vi "Activate ECL Guest Internet (SubVI).vi"(0 "Status String Ref":refnum<vi>, 7 "Activate":bool, 11 "Error IN":errorcluster, 14 "Ok to Click?":bool) -> (15 "Error OUT":errorcluster)   [LabVIEW 2012]
panel:
  in  "Web Browser":refnum<k7>(container)
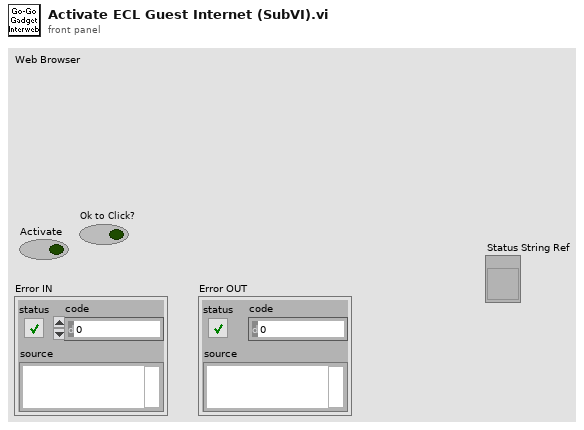
[diagram p1: front panel]
types:
  T1 = enum16{"Initialize", "Wait for Authorize Page", "Click Authorize", "Idle", "Exit"}
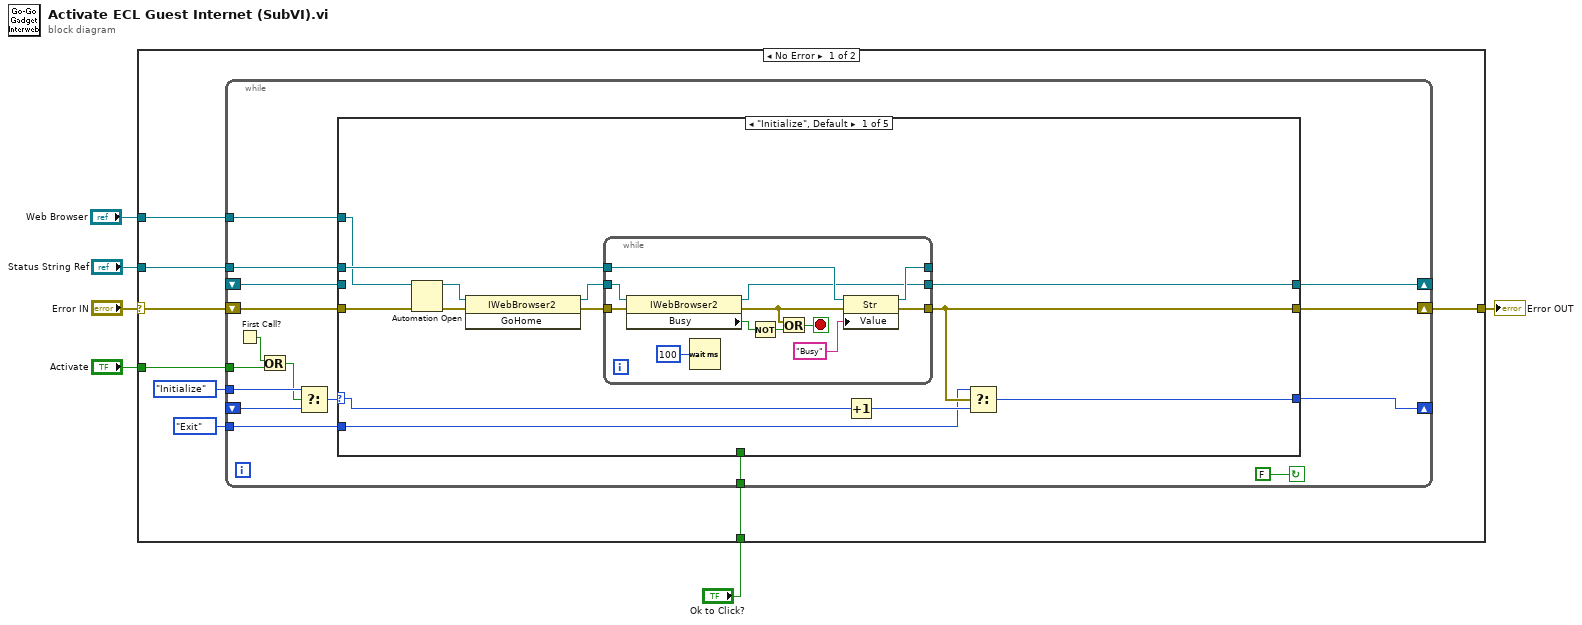
[diagram p0: block diagram]
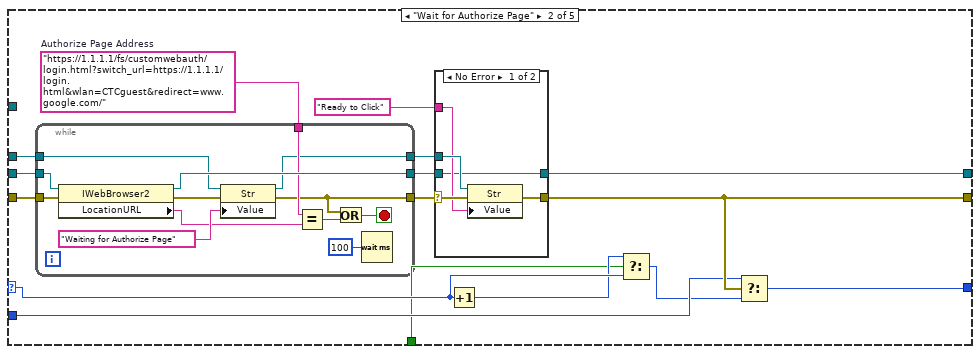
[diagram p2: hidden frame]
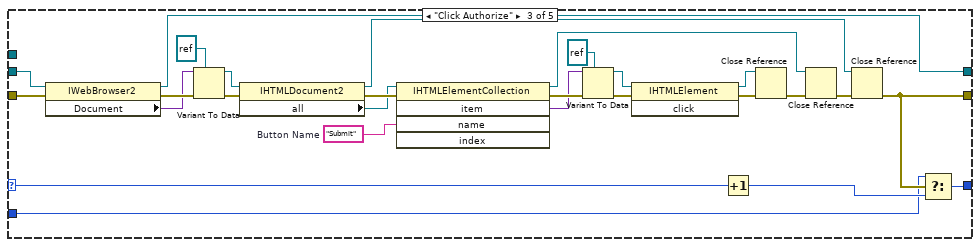
[diagram p4: hidden frame]
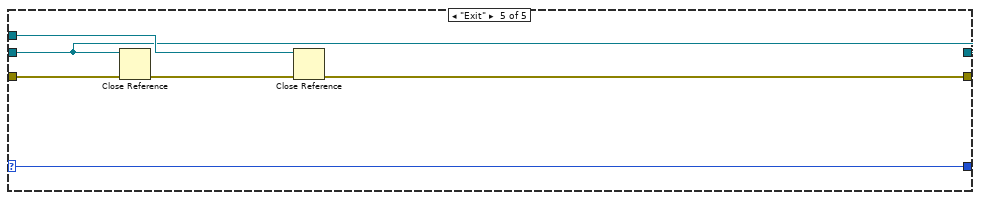
[diagram p6: hidden frame]
diagram:
  n1 = case shown="No Error" "Error IN" {
    selector: "Error IN" -> [w9 w128]
    tunnel: "Status String Ref" -> [w14 _]
    tunnel: "Activate" -> [w11 _]
    tunnel: [w10 w128] -> w4
    tunnel: "Web Browser" -> [w8 _]
    tunnel: "Ok to Click?" -> [w7 _]
    frame No Error {
      n2 = while {
        shift-right: [w29] -> _
        shift-left: _ -> [w28]
        shift-right: [w25] -> w10
        shift-left: w9 -> [w27]
        tunnel: w14 -> [w26]
        shift-right: [w21] -> _
        shift-left: _ -> [w23]
        tunnel: T1."Initialize" ("State") -> [w24]
        tunnel: T1."Exit" ("State") -> [w20]
        tunnel: w11 -> [w19]
        tunnel: w8 -> [w16]
        tunnel: w7 -> [w15]
        stop <- FALSE continue-if-true
        n3 = First Call?() -> (First Call?: T/F=w18:bool)
        n4 = Or(x=w18, y=w19) -> (x .or. y?=w17:bool)
        n5 = Select(t=w24, s=w17, f=w23) -> (s? t:f=w22:T1)
        n6 = case shown="\"Initialize\", Default" w22 {
          selector: w22 -> [w35 w59 w115 w121 w123]
          tunnel: [w37 w63 w116 w119 w122] -> w29
          tunnel: w28 -> [_ w70 w117 w119 w122]
          tunnel: w27 -> [w38 w71 w118 w120 w127]
          tunnel: w26 -> [w41 w69 _ _ w126]
          tunnel: [w36 w62 w113 w120 w124] -> w25
          tunnel: [w33 w60 w114 w121 w123] -> w21
          tunnel: w20 -> [w32 w61 w92 _ _]
          tunnel: w16 -> [w31 _ _ _ _]
          tunnel: w15 -> [_ w56 _ _ _]
          frame "Initialize", Default {
            n7 = Automation Open(error in (no error)=w38, Automation Refnum=w31) -> (Automation Refnum=w40:refnum<k7>, error out=w43:errorcluster)  [unwired: 2 in]
            n8 = invoke class="IWebBrowser2" method="GoHome"(reference=w40, error in=w43) -> (reference out=w39:refnum<k7>, error out=w42:errorcluster)  [unwired: 1 in, 1 out]
            n9 = while {
              tunnel: [w49] -> w36
              tunnel: w42 -> [w52]
              tunnel: w41 -> [w51]
              tunnel: [w48] -> _
              tunnel: w39 -> [w44]
              tunnel: [w47] -> w37
              stop <- w55 stop-if-true
              n10 = property class="IWebBrowser2"(reference=w44, error in=w52) -> (reference out=w47:refnum<k7>, error out=w45:errorcluster, "Busy"=w53:bool)
              n11 = Wait (ms)(milliseconds to wait=u32 100) -> ()  [unwired: 1 out]
              n12 = Not(x=w53) -> (.not. x?=w46:bool)
              n13 = Or(x=w45, y=w46) -> (x .or. y?=w55:bool)
              n14 = property class="Str"(reference=w51, error in=w45, "Value"="Busy") -> (reference out=w48:refnum<vi>, error out=w49:errorcluster)
            }
            n15 = Increment(x=w35) -> (x+1=w34:T1)
            n16 = Select(t=w32, s=w36, f=w34) -> (s? t:f=w33:T1)
          }
          frame "Wait for Authorize Page" {
            w68 = "https://1.1.1.1/fs/customwebauth/login.html?switch_url=https://1.1.1.1/login.html&wlan=CTCguest&redirect=www.google.com/"  # Authorize Page Address
            n17 = while {
              tunnel: w71 -> [w91]
              tunnel: w69 -> [w80]
              tunnel: w68 -> [w85]
              tunnel: w70 -> [w87]
              tunnel: [w86] -> w66
              tunnel: [w81] -> w67
              tunnel: [w79] -> w65
              stop <- w82 stop-if-true
              n18 = property class="IWebBrowser2"(reference=w87, error in=w91) -> (reference out=w86:refnum<k7>, error out=w90:errorcluster, "LocationURL"=w84:string)
              n19 = property class="Str"(reference=w80, error in=w90, "Value"="Waiting for Authorize Page") -> (reference out=w79:refnum<vi>, error out=w81:errorcluster)
              n20 = Equal?(x=w85, y=w84) -> (x = y?=w83:bool)
              n21 = Or(x=w81, y=w83) -> (x .or. y?=w82:bool)
              n22 = Wait (ms)(milliseconds to wait=u32 100) -> ()  [unwired: 1 out]
            }
            n23 = case shown="No Error" w67 {
              selector: w67 -> [w76 w77]
              tunnel: w66 -> [w72 w78]
              tunnel: w65 -> [w75 _]
              tunnel: "Ready to Click" ("Value") -> [w74 _]
              tunnel: [w73 w77] -> w62
              tunnel: [w72 w78] -> w63
              frame No Error {
                n24 = property class="Str"(reference=w75, error in=w76, "Value"=w74) -> (error out=w73:errorcluster)  [unwired: 1 out]
              }
              frame Error {
              }
            }
            n25 = Increment(x=w59) -> (x+1=w58:T1)
            n26 = Select(t=w58, s=w56, f=w59) -> (s? t:f=w57:T1)
            n27 = Select(t=w61, s=w62, f=w57) -> (s? t:f=w60:T1)
          }
          frame "Click Authorize" {
            w108 = "Submit"  # Button Name
            n28 = property class="IWebBrowser2"(reference=w117, error in=w118) -> (reference out=w116:refnum<k7>, error out=w98:errorcluster, "Document"=w97:variant)
            n29 = Variant To Data(error in=w98, type=refnum<k7> refnum ("MSHTML.IHTMLDocument2"), Variant=w97) -> (data=w100:refnum<k7>, error out=w99:errorcluster)
            n30 = property class="IHTMLDocument2"(reference=w100, error in=w99) -> (reference out=w94:refnum<k7>, error out=w96:errorcluster, "all"=w95:refnum<k7>)
            n31 = invoke class="IHTMLElementCollection" method="item"(reference=w95, error in=w96, "name"=w108) -> (reference out=w105:refnum<k7>, error out=w111:errorcluster, "item"=w109:variant)  [unwired: 2 in, 2 out]
            n32 = Variant To Data(error in=w111, type=refnum<k7> refnum ("MSHTML.IHTMLElement"), Variant=w109) -> (data=w110:refnum<k7>, error out=w112:errorcluster)
            n33 = invoke class="IHTMLElement" method="click"(reference=w110, error in=w112) -> (reference out=w107:refnum<k7>, error out=w106:errorcluster)  [unwired: 1 in, 1 out]
            n34 = Increment(x=w115) -> (x+1=w93:T1)
            n35 = Close Reference(reference=w107, error in (no error)=w106) -> (error out=w104:errorcluster)
            n36 = Close Reference(reference=w105, error in (no error)=w104) -> (error out=w103:errorcluster)
            n37 = Close Reference(reference=w94, error in (no error)=w103) -> (error out=w113:errorcluster)
            n38 = Select(t=w92, s=w113, f=w93) -> (s? t:f=w114:T1)
          }
          frame "Idle" {
          }
          frame "Exit" {
            n39 = Close Reference(reference=w122, error in (no error)=w127) -> (error out=w125:errorcluster)
            n40 = Close Reference(reference=w126, error in (no error)=w125) -> (error out=w124:errorcluster)
          }
        }
      }
    }
    frame Error {
    }
  }
  "Error OUT" <- w4
